vi "Version_4.9_8_on-chip_valves_for25ulSyringe_withModfied_Plunging.vi"() -> ()   [LabVIEW 2020] (continued)
                                n2256 = call "RPickUp(SubVI).vi"("Volume to be picked up"=w2683, "Volume of Syringe"=w2686, "Resolution of PickUP"=w2684, "PickUp Flow Rate (ul/min)"=w2685, "VISA Refnum in"=w2687) -> ()  [unwired: 6 in, 1 out]
                                }
                                frame #1 {
                                n2257 = while {
                                stop <- w2688 stop-if-true
                                n2258 = local read "Stopper that ends \nthe main loops"() -> (w2689:bool)
                                n2259 = local read "VISA Refnum in\nfor Pump"() -> (w2690:refnum<visa-resource-name>)
                                n2260 = case shown="True" w2689 {
                                frame False {
                                }
                                frame True {
                                n2261 = local read "VISA Refnum in\nfor Pump"() -> (w2691:refnum<visa-resource-name>)
                                n2262 = call "HardStopCurrentProcess (SubVI).vi"("VISA Refnum in"=w2691) -> ()  [unwired: 11 in]
                                }
                                }
                                n2263 = call "ProcessCompletionWaiterWithOutPut (SubVI).vi"("VISA Refnum in"=w2690) -> ("Boolean"=w2688:bool)  [unwired: 10 in]
                                }
                                }
                                frame #2 {
                                # "Reads the initial Plunger Position for computing the volume dispensed"
                                n2264 = local read "VISA Refnum in\nfor Pump"() -> (w2693:refnum<visa-resource-name>)
                                n2265 = call "AbsolutePlungerPosition (SubVI).vi"("VISA Refnum in"=w2693) -> ("Plunger Position"=w2692:i32)  [unwired: 10 in]
                                n2266 = local write "Initial Plunger Position"(w2692) -> ()
                                }
                                frame #3 {
                                # "Switch to Port-2"
                                # "Port-2 of the pump is conncted to column-1 of chip"
                                n2267 = local read "VISA Refnum in\nfor Pump"() -> (w2695:refnum<visa-resource-name>)
                                n2268 = call "PortChanger (SubVI).vi"("Port Number"="2", "VISA Refnum in"=w2695) -> ()  [unwired: 10 in]
                                }
                                frame #4 {
                                n2269 = while {
                                stop <- w2696 stop-if-true
                                n2270 = local read "Stopper that ends \nthe main loops"() -> (w2697:bool)
                                n2271 = local read "VISA Refnum in\nfor Pump"() -> (w2698:refnum<visa-resource-name>)
                                n2272 = case shown="True" w2697 {
                                frame False {
                                }
                                frame True {
                                n2273 = local read "VISA Refnum in\nfor Pump"() -> (w2699:refnum<visa-resource-name>)
                                n2274 = call "HardStopCurrentProcess (SubVI).vi"("VISA Refnum in"=w2699) -> ()  [unwired: 11 in]
                                }
                                }
                                n2275 = call "ProcessCompletionWaiterWithOutPut (SubVI).vi"("VISA Refnum in"=w2698) -> ("Boolean"=w2696:bool)  [unwired: 10 in]
                                }
                                }
                                frame #5 {
                                n2276 = local read "Buffer-A1 Dispense\nFlow Rate (ul/min) \nfor Equilibration\nof Column-1"() -> (w2703:dbl)
                                n2277 = local read "Buffer-A1 Pumping\nResolution \nfor Equilibration \nof Column-1"() -> (w2702:T2)
                                n2278 = local read "VISA Refnum in\nfor Pump"() -> (w2705:refnum<visa-resource-name>)
                                n2279 = local write "Pause Data Collection"(FALSE ("Pause Data Collection")) -> ()
                                n2280 = local read "Volume of Syringe"() -> (w2704:dbl)
                                n2281 = call "GoToAbsolutePosition(SubVI).vi"("Absolute Volume Position in Syringe (in ul)"=0.0, "Volume of Syringe"=w2704, "Resolution of Pumping"=w2702, "Flow Rate (ul/min)"=w2703, "VISA Refnum in"=w2705) -> ()  [unwired: 6 in, 1 out]
                                }
                                frame #6 {
                                n2282 = local read "Buffer-A1 Pumping\nResolution \nfor Equilibration \nof Column-1"() -> (w2707:T2)
                                n2283 = local read "VISA Refnum in\nfor Pump"() -> (w2709:refnum<visa-resource-name>)
                                n2284 = local read "Initial Plunger Position"() -> (w2708:dbl)
                                n2285 = local read "Volume of Syringe"() -> (w2706:dbl)
                                n2286 = while {
                                tunnel: w2708 -> [w2716]
                                tunnel: w2709 -> [w2715]
                                tunnel: w2707 -> [w2714]
                                tunnel: w2706 -> [w2713]
                                stop <- w2711 stop-if-true
                                n2287 = stacked-sequence {
                                tunnel: w2716 -> [w2723 _]
                                tunnel: w2715 -> [w2722 w2743]
                                tunnel: w2714 -> [w2721 _]
                                tunnel: w2713 -> [w2720 _]
                                tunnel: [_ w2741] -> w2711
                                frame #0 {
                                n2288 = call "AbsolutePlungerPosition (SubVI).vi"("VISA Refnum in"=w2722) -> ("Plunger Position"=w2719:i32)  [unwired: 10 in]
                                n2289 = case shown="\"Standard Pumping\", Default" w2721 {
                                tunnel: w2723 -> [w2728 w2737]
                                tunnel: w2719 -> [w2729 w2736]
                                tunnel: [w2727 w2734] -> w2718
                                tunnel: w2720 -> [w2726 w2735]
                                frame "Standard Pumping", Default {
                                n2290 = Subtract(x=w2728, y=w2729) -> (x-y=w2725:dbl)
                                n2291 = Absolute Value(x=w2725) -> (abs(x)=w2724:dbl)
                                n2292 = Multiply(x=w2724, y=w2726) -> (x*y=w2731:dbl)
                                n2293 = Divide(x=w2731, y=3000.0) -> (x/y=w2727:dbl)
                                }
                                frame "High Resolution Pumping" {
                                n2294 = Subtract(x=w2737, y=w2736) -> (x-y=w2733:dbl)
                                n2295 = Absolute Value(x=w2733) -> (abs(x)=w2732:dbl)
                                n2296 = Multiply(x=w2732, y=w2735) -> (x*y=w2739:dbl)
                                n2297 = Divide(x=w2739, y=24000.0) -> (x/y=w2734:dbl)
                                }
                                }
                                n2298 = local write "Volume being Injected \nin this process"(w2718) -> ()
                                }
                                frame #1 {
                                n2299 = call "LSPOneStatus (SubVI).vi"("VISA Refnum in"=w2743) -> ("read buffer"=w2745:string)  [unwired: 10 in]
                                n2300 = call <vilib>:"Trim Whitespace.vi"("string"=w2745) -> ("trimmed string"=w2744:string)  [unwired: 1 in]
                                n2301 = local read "Stopper that ends \nthe main loops"() -> (w2740:bool)
                                n2302 = Equal?(x=w2744, y="/0`\u0003") -> (x = y?=w2742:bool)
                                n2303 = Or(x=w2742, y=w2740) -> (x .or. y?=w2741:bool)
                                }
                                }
                                n2304 = Wait (ms)(milliseconds to wait=u32 100) -> ()  [unwired: 1 out]
                                n2305 = local read "Stopper that ends \nthe main loops"() -> (w2710:bool)
                                n2306 = case shown="True" w2710 {
                                frame False {
                                }
                                frame True {
                                n2307 = local read "VISA Refnum in\nfor Pump"() -> (w2717:refnum<visa-resource-name>)
                                n2308 = call "HardStopCurrentProcess (SubVI).vi"("VISA Refnum in"=w2717) -> ()  [unwired: 11 in]
                                }
                                }
                                }
                                }
                                frame #7 {
                                # "Change the pump port back to Buffer-A1"
                                n2309 = local read "VISA Refnum in\nfor Pump"() -> (w2748:refnum<visa-resource-name>)
                                n2310 = local read "Port for \nA1-Equilibriation"() -> (w2747:string)
                                n2311 = local write "Pause Data Collection"(TRUE ("Pause Data Collection")) -> ()
                                n2312 = Wait (ms)(milliseconds to wait=u32 500) -> ()  [unwired: 1 out]
                                n2313 = call "PortChanger (SubVI).vi"("Port Number"=w2747, "VISA Refnum in"=w2748) -> ()  [unwired: 10 in]
                                }
                                frame #8 {
                                n2314 = local read "VISA Refnum in\nfor Pump"() -> (w2751:refnum<visa-resource-name>)
                                n2315 = local write "Volume being Injected \nin this process"(0.0 ("Volume being Injected \nin this process")) -> ()
                                n2316 = call "ProcessCompletionWaiter (SubVI).vi"("VISA Refnum in"=w2751) -> ()  [unwired: 11 in]
                                }
                              }
                            }
                            n2317 = local write "Reminder of the \nVolume to be \nPumped"(w2680) -> ()
                          }
                          frame #6 {
                            n2318 = stacked-sequence {
                              frame #0 {
                                n2319 = local read "Buffer-A1 PickUp \nFlow Rate (ul/min)\nfor Equilibration \nof Column-1"() -> (w2755:dbl)
                                n2320 = local read "Buffer-A1 Pumping\nResolution \nfor Equilibration \nof Column-1"() -> (w2754:T2)
                                n2321 = local read "VISA Refnum in\nfor Pump"() -> (w2757:refnum<visa-resource-name>)
                                n2322 = local read "Reminder of the \nVolume to be \nPumped"() -> (w2753:dbl)
                                n2323 = local read "Volume of Syringe"() -> (w2756:dbl)
                                n2324 = call "RPickUp(SubVI).vi"("Volume to be picked up"=w2753, "Volume of Syringe"=w2756, "Resolution of PickUP"=w2754, "PickUp Flow Rate (ul/min)"=w2755, "VISA Refnum in"=w2757) -> ()  [unwired: 6 in, 1 out]
                              }
                              frame #1 {
                                n2325 = while {
                                stop <- w2758 stop-if-true
                                n2326 = local read "Stopper that ends \nthe main loops"() -> (w2759:bool)
                                n2327 = local read "VISA Refnum in\nfor Pump"() -> (w2760:refnum<visa-resource-name>)
                                n2328 = case shown="True" w2759 {
                                frame False {
                                }
                                frame True {
                                n2329 = local read "VISA Refnum in\nfor Pump"() -> (w2761:refnum<visa-resource-name>)
                                n2330 = call "HardStopCurrentProcess (SubVI).vi"("VISA Refnum in"=w2761) -> ()  [unwired: 11 in]
                                }
                                }
                                n2331 = call "ProcessCompletionWaiterWithOutPut (SubVI).vi"("VISA Refnum in"=w2760) -> ("Boolean"=w2758:bool)  [unwired: 10 in]
                                }
                              }
                              frame #2 {
                                # "Reads the initial Plunger Position for computing the volume dispensed"
                                n2332 = local read "VISA Refnum in\nfor Pump"() -> (w2763:refnum<visa-resource-name>)
                                n2333 = call "AbsolutePlungerPosition (SubVI).vi"("VISA Refnum in"=w2763) -> ("Plunger Position"=w2762:i32)  [unwired: 10 in]
                                n2334 = local write "Initial Plunger Position"(w2762) -> ()
                              }
                              frame #3 {
                                # "Switch to Port-2"
                                # "Port-2 of the pump is conncted to column-1 of chip"
                                n2335 = local read "VISA Refnum in\nfor Pump"() -> (w2765:refnum<visa-resource-name>)
                                n2336 = call "PortChanger (SubVI).vi"("Port Number"="2", "VISA Refnum in"=w2765) -> ()  [unwired: 10 in]
                              }
                              frame #4 {
                                n2337 = while {
                                stop <- w2766 stop-if-true
                                n2338 = local read "Stopper that ends \nthe main loops"() -> (w2767:bool)
                                n2339 = local read "VISA Refnum in\nfor Pump"() -> (w2768:refnum<visa-resource-name>)
                                n2340 = case shown="True" w2767 {
                                frame False {
                                }
                                frame True {
                                n2341 = local read "VISA Refnum in\nfor Pump"() -> (w2769:refnum<visa-resource-name>)
                                n2342 = call "HardStopCurrentProcess (SubVI).vi"("VISA Refnum in"=w2769) -> ()  [unwired: 11 in]
                                }
                                }
                                n2343 = call "ProcessCompletionWaiterWithOutPut (SubVI).vi"("VISA Refnum in"=w2768) -> ("Boolean"=w2766:bool)  [unwired: 10 in]
                                }
                              }
                              frame #5 {
                                n2344 = local read "Buffer-A1 Pumping\nResolution \nfor Equilibration \nof Column-1"() -> (w2772:T2)
                                n2345 = local read "Buffer-A1 Dispense\nFlow Rate (ul/min) \nfor Equilibration\nof Column-1"() -> (w2773:dbl)
                                n2346 = local read "VISA Refnum in\nfor Pump"() -> (w2775:refnum<visa-resource-name>)
                                n2347 = local write "Pause Data Collection"(FALSE ("Pause Data Collection")) -> ()
                                n2348 = local read "Volume of Syringe"() -> (w2774:dbl)
                                n2349 = call "GoToAbsolutePosition(SubVI).vi"("Absolute Volume Position in Syringe (in ul)"=0.0 ("Volume to be Dispensed"), "Volume of Syringe"=w2774, "Resolution of Pumping"=w2772, "Flow Rate (ul/min)"=w2773, "VISA Refnum in"=w2775) -> ()  [unwired: 6 in, 1 out]
                              }
                              frame #6 {
                                n2350 = local read "Buffer-A1 Pumping\nResolution \nfor Equilibration \nof Column-1"() -> (w2777:T2)
                                n2351 = local read "VISA Refnum in\nfor Pump"() -> (w2779:refnum<visa-resource-name>)
                                n2352 = local read "Initial Plunger Position"() -> (w2778:dbl)
                                n2353 = local read "Volume of Syringe"() -> (w2776:dbl)
                                n2354 = while {
                                tunnel: w2778 -> [w2786]
                                tunnel: w2779 -> [w2785]
                                tunnel: w2777 -> [w2784]
                                tunnel: w2776 -> [w2783]
                                stop <- w2781 stop-if-true
                                n2355 = stacked-sequence {
                                tunnel: w2786 -> [w2793 _]
                                tunnel: w2785 -> [w2792 w2813]
                                tunnel: w2784 -> [w2791 _]
                                tunnel: w2783 -> [w2790 _]
                                tunnel: [_ w2811] -> w2781
                                frame #0 {
                                n2356 = call "AbsolutePlungerPosition (SubVI).vi"("VISA Refnum in"=w2792) -> ("Plunger Position"=w2789:i32)  [unwired: 10 in]
                                n2357 = case shown="\"Standard Pumping\", Default" w2791 {
                                tunnel: w2793 -> [w2798 w2807]
                                tunnel: w2789 -> [w2799 w2806]
                                tunnel: [w2797 w2804] -> w2788
                                tunnel: w2790 -> [w2796 w2805]
                                frame "Standard Pumping", Default {
                                n2358 = Subtract(x=w2798, y=w2799) -> (x-y=w2795:dbl)
                                n2359 = Absolute Value(x=w2795) -> (abs(x)=w2794:dbl)
                                n2360 = Multiply(x=w2794, y=w2796) -> (x*y=w2801:dbl)
                                n2361 = Divide(x=w2801, y=3000.0) -> (x/y=w2797:dbl)
                                }
                                frame "High Resolution Pumping" {
                                n2362 = Subtract(x=w2807, y=w2806) -> (x-y=w2803:dbl)
                                n2363 = Absolute Value(x=w2803) -> (abs(x)=w2802:dbl)
                                n2364 = Multiply(x=w2802, y=w2805) -> (x*y=w2809:dbl)
                                n2365 = Divide(x=w2809, y=24000.0) -> (x/y=w2804:dbl)
                                }
                                }
                                n2366 = local write "Volume being Injected \nin this process"(w2788) -> ()
                                }
                                frame #1 {
                                n2367 = call "LSPOneStatus (SubVI).vi"("VISA Refnum in"=w2813) -> ("read buffer"=w2815:string)  [unwired: 10 in]
                                n2368 = call <vilib>:"Trim Whitespace.vi"("string"=w2815) -> ("trimmed string"=w2814:string)  [unwired: 1 in]
                                n2369 = local read "Stopper that ends \nthe main loops"() -> (w2810:bool)
                                n2370 = Equal?(x=w2814, y="/0`\u0003") -> (x = y?=w2812:bool)
                                n2371 = Or(x=w2812, y=w2810) -> (x .or. y?=w2811:bool)
                                }
                                }
                                n2372 = Wait (ms)(milliseconds to wait=u32 100) -> ()  [unwired: 1 out]
                                n2373 = local read "Stopper that ends \nthe main loops"() -> (w2780:bool)
                                n2374 = case shown="True" w2780 {
                                frame False {
                                }
                                frame True {
                                n2375 = local read "VISA Refnum in\nfor Pump"() -> (w2787:refnum<visa-resource-name>)
                                n2376 = call "HardStopCurrentProcess (SubVI).vi"("VISA Refnum in"=w2787) -> ()  [unwired: 11 in]
                                }
                                }
                                }
                              }
                              frame #7 {
                                # "Change the pump port to Buffer-C1 for equilibriation of column-2"
                                n2377 = local read "VISA Refnum in\nfor Pump"() -> (w2818:refnum<visa-resource-name>)
                                n2378 = local read "Port for \nC1-Equilibriation"() -> (w2817:string)
                                n2379 = local write "Pause Data Collection"(TRUE ("Pause Data Collection")) -> ()
                                n2380 = Wait (ms)(milliseconds to wait=u32 500) -> ()  [unwired: 1 out]
                                n2381 = call "PortChanger (SubVI).vi"("Port Number"=w2817, "VISA Refnum in"=w2818) -> ()  [unwired: 10 in]
                              }
                              frame #8 {
                                n2382 = local read "VISA Refnum in\nfor Pump"() -> (w2822:refnum<visa-resource-name>)
                                n2383 = local write "Volume being Injected \nin this process"(0.0 ("Volume being Injected \nin this process")) -> ()
                                n2384 = call "ProcessCompletionWaiter (SubVI).vi"("VISA Refnum in"=w2822) -> ()  [unwired: 11 in]
                                n2385 = local write "Start the Process"(FALSE ("Start the Process")) -> ()
                              }
                            }
                          }
                          frame #7 {
                            # "Clean the tubing with Buffer-C1"
                            n2386 = local read "N-C1"() -> (w2825:i32)
                            n2387 = local write "Equilibriating \nColumn-1"(FALSE ("Equilibriating \nColumn-1")) -> ()
                            n2388 = for {
                              N: w2825 -> [_]
                              n2389 = stacked-sequence {
                                frame #0 {
                                n2390 = local read "Port for \nC1-Equilibriation"() -> (w2828:string)
                                n2391 = local read "VISA Refnum in\nfor Pump"() -> (w2829:refnum<visa-resource-name>)
                                n2392 = call "PortChanger (SubVI).vi"("Port Number"=w2828, "VISA Refnum in"=w2829) -> ()  [unwired: 10 in]
                                }
                                frame #1 {
                                n2393 = local read "VISA Refnum in\nfor Pump"() -> (w2830:refnum<visa-resource-name>)
                                n2394 = call "ProcessCompletionWaiter (SubVI).vi"("VISA Refnum in"=w2830) -> ()  [unwired: 11 in]
                                }
                                frame #2 {
                                n2395 = local read "VISA Refnum in\nfor Pump"() -> (w2835:refnum<visa-resource-name>)
                                n2396 = local read "Apparent Volume\nof Syringe"() -> (w2831:dbl)
                                n2397 = local read "Volume of Syringe"() -> (w2832:dbl)
                                n2398 = call "RPickUp(SubVI).vi"("Volume to be picked up"=w2831, "Volume of Syringe"=w2832, "Resolution of PickUP"=T2."Standard Pumping", "PickUp Flow Rate (ul/min)"=150.0, "VISA Refnum in"=w2835) -> ()  [unwired: 6 in, 1 out]
                                }
                                frame #3 {
                                n2399 = local read "Stopper that ends \nthe main loops"() -> (w2836:bool)
                                n2400 = local read "VISA Refnum in\nfor Pump"() -> (w2837:refnum<visa-resource-name>)
                                n2401 = case shown="True" w2836 {
                                frame False {
                                }
                                frame True {
                                n2402 = local read "VISA Refnum in\nfor Pump"() -> (w2838:refnum<visa-resource-name>)
                                n2403 = call "HardStopCurrentProcess (SubVI).vi"("VISA Refnum in"=w2838) -> ()  [unwired: 11 in]
                                }
                                }
                                n2404 = call "ProcessCompletionWaiter (SubVI).vi"("VISA Refnum in"=w2837) -> ()  [unwired: 11 in]
                                }
                                frame #4 {
                                n2405 = local read "VISA Refnum in\nfor Pump"() -> (w2840:refnum<visa-resource-name>)
                                n2406 = call "PortChanger (SubVI).vi"("Port Number"="1", "VISA Refnum in"=w2840) -> ()  [unwired: 10 in]
                                }
                                frame #5 {
                                n2407 = local read "Stopper that ends \nthe main loops"() -> (w2841:bool)
                                n2408 = local read "VISA Refnum in\nfor Pump"() -> (w2842:refnum<visa-resource-name>)
                                n2409 = case shown="True" w2841 {
                                frame False {
                                }
                                frame True {
                                n2410 = local read "VISA Refnum in\nfor Pump"() -> (w2843:refnum<visa-resource-name>)
                                n2411 = call "HardStopCurrentProcess (SubVI).vi"("VISA Refnum in"=w2843) -> ()  [unwired: 11 in]
                                }
                                }
                                n2412 = call "ProcessCompletionWaiter (SubVI).vi"("VISA Refnum in"=w2842) -> ()  [unwired: 11 in]
                                }
                                frame #6 {
                                n2413 = local read "VISA Refnum in\nfor Pump"() -> (w2848:refnum<visa-resource-name>)
                                n2414 = local read "Volume of Syringe"() -> (w2845:dbl)
                                n2415 = call "GoToAbsolutePosition(SubVI).vi"("Absolute Volume Position in Syringe (in ul)"=0.0 ("Volume to be picked up"), "Volume of Syringe"=w2845, "Resolution of Pumping"=T2."Standard Pumping" ("Resolution of PickUP"), "Flow Rate (ul/min)"=150.0 ("PickUp Flow Rate (ul/min)"), "VISA Refnum in"=w2848) -> ()  [unwired: 6 in, 1 out]
                                }
                                frame #7 {
                                n2416 = local read "Stopper that ends \nthe main loops"() -> (w2849:bool)
                                n2417 = local read "VISA Refnum in\nfor Pump"() -> (w2850:refnum<visa-resource-name>)
                                n2418 = case shown="True" w2849 {
                                frame False {
                                }
                                frame True {
                                n2419 = local read "VISA Refnum in\nfor Pump"() -> (w2851:refnum<visa-resource-name>)
                                n2420 = call "HardStopCurrentProcess (SubVI).vi"("VISA Refnum in"=w2851) -> ()  [unwired: 11 in]
                                }
                                }
                                n2421 = call "ProcessCompletionWaiter (SubVI).vi"("VISA Refnum in"=w2850) -> ()  [unwired: 11 in]
                                }
                              }
                            }
                            n2422 = local write "Pause Data Collection"(TRUE ("Pause Data Collection")) -> ()
                            n2423 = local write "Equilibriating \nColumn-2"(TRUE ("Equilibriating \nColumn-2")) -> ()
                          }
                          frame #8 {
                            n2424 = local read "Buffer-C1 Volume \nto be  Pumped \nfor Equilibration\nof Column-2"() -> (w2855:dbl)
                            n2425 = local read "Apparent Volume\nof Syringe"() -> (w2852:dbl)
                            n2426 = Quotient & Remainder(x=w2855, y=w2852) -> (x-y*floor(x/y)=w2853:dbl, floor(x/y)=w2854:dbl)
                            n2427 = for {
                              N: w2854 -> [_]
                              n2428 = stacked-sequence {
                                frame #0 {
                                n2429 = local read "VISA Refnum in\nfor Pump"() -> (w2857:refnum<visa-resource-name>)
                                n2430 = local read "Port for \nC1-Equilibriation"() -> (w2856:string)
                                n2431 = call "PortChanger (SubVI).vi"("Port Number"=w2856, "VISA Refnum in"=w2857) -> ()  [unwired: 10 in]
                                }
                                frame #1 {
                                n2432 = local read "VISA Refnum in\nfor Pump"() -> (w2858:refnum<visa-resource-name>)
                                n2433 = call "ProcessCompletionWaiter (SubVI).vi"("VISA Refnum in"=w2858) -> ()  [unwired: 11 in]
                                }
                                frame #2 {
                                n2434 = local read "Buffer-C1 PickUp \nFlow Rate (ul/min)\nfor Equilibration \nof Column-2"() -> (w2861:dbl)
                                n2435 = local read "Buffer-C1 Pumping\nResolution \nfor Equilibration \nof Column-2"() -> (w2860:T2)
                                n2436 = local read "VISA Refnum in\nfor Pump"() -> (w2863:refnum<visa-resource-name>)
                                n2437 = local read "Apparent Volume\nof Syringe"() -> (w2859:dbl)
                                n2438 = local read "Volume of Syringe"() -> (w2862:dbl)
                                n2439 = call "RPickUp(SubVI).vi"("Volume to be picked up"=w2859, "Volume of Syringe"=w2862, "Resolution of PickUP"=w2860, "PickUp Flow Rate (ul/min)"=w2861, "VISA Refnum in"=w2863) -> ()  [unwired: 6 in, 1 out]
                                }
                                frame #3 {
                                n2440 = while {
                                stop <- w2864 stop-if-true
                                n2441 = local read "Stopper that ends \nthe main loops"() -> (w2865:bool)
                                n2442 = local read "VISA Refnum in\nfor Pump"() -> (w2866:refnum<visa-resource-name>)
                                n2443 = case shown="True" w2865 {
                                frame False {
                                }
                                frame True {
                                n2444 = local read "VISA Refnum in\nfor Pump"() -> (w2867:refnum<visa-resource-name>)
                                n2445 = call "HardStopCurrentProcess (SubVI).vi"("VISA Refnum in"=w2867) -> ()  [unwired: 11 in]
                                }
                                }
                                n2446 = call "ProcessCompletionWaiterWithOutPut (SubVI).vi"("VISA Refnum in"=w2866) -> ("Boolean"=w2864:bool)  [unwired: 10 in]
                                }
                                }
                                frame #4 {
                                # "Reads the initial Plunger Position for computing the volume dispensed"
                                n2447 = local read "VISA Refnum in\nfor Pump"() -> (w2869:refnum<visa-resource-name>)
                                n2448 = call "AbsolutePlungerPosition (SubVI).vi"("VISA Refnum in"=w2869) -> ("Plunger Position"=w2868:i32)  [unwired: 10 in]
                                n2449 = local write "Initial Plunger Position"(w2868) -> ()
                                }
                                frame #5 {
                                # "Switch to Port-10"
                                # "Port-10 of the pump is conncted to column-2 of chip"
                                n2450 = local read "VISA Refnum in\nfor Pump"() -> (w2871:refnum<visa-resource-name>)
                                n2451 = call "PortChanger (SubVI).vi"("Port Number"="10", "VISA Refnum in"=w2871) -> ()  [unwired: 10 in]
                                }
                                frame #6 {
                                n2452 = while {
                                stop <- w2872 stop-if-true
                                n2453 = local read "Stopper that ends \nthe main loops"() -> (w2873:bool)
                                n2454 = local read "VISA Refnum in\nfor Pump"() -> (w2874:refnum<visa-resource-name>)
                                n2455 = case shown="True" w2873 {
                                frame False {
                                }
                                frame True {
                                n2456 = local read "VISA Refnum in\nfor Pump"() -> (w2875:refnum<visa-resource-name>)
                                n2457 = call "HardStopCurrentProcess (SubVI).vi"("VISA Refnum in"=w2875) -> ()  [unwired: 11 in]
                                }
                                }
                                n2458 = call "ProcessCompletionWaiterWithOutPut (SubVI).vi"("VISA Refnum in"=w2874) -> ("Boolean"=w2872:bool)  [unwired: 10 in]
                                }
                                }
                                frame #7 {
                                # "Buffer-C pumped for column non-interference"
                                # "Keeps the AMF valve after column-1 open and valve after column-2 closed"
                                n2459 = local read "Buffer-C1 Dispense\nFlow Rate (ul/min) \nfor Equilibration\nof Column-2"() -> (w2888:dbl)
                                n2460 = local read "Buffer-C1 Pumping\nResolution \nfor Equilibration \nof Column-2"() -> (w2887:T2)
                                n2461 = local read "VISA Refnum in\nfor Pump"() -> (w2890:refnum<visa-resource-name>)
                                n2462 = local write "Pause Data Collection"(FALSE ("Pause Data Collection")) -> ()
                                n2463 = local read "Volume of Syringe"() -> (w2889:dbl)
                                n2464 = call "GoToAbsolutePosition(SubVI).vi"("Absolute Volume Position in Syringe (in ul)"=0.0, "Volume of Syringe"=w2889, "Resolution of Pumping"=w2887, "Flow Rate (ul/min)"=w2888, "VISA Refnum in"=w2890) -> ()  [unwired: 6 in, 1 out]
                                n2465 = local write "Valve V1 Open"(FALSE ("Valve V1 Open")) -> ()
                                n2466 = local write "Valve V2 Open"(TRUE ("Valve V2 Open")) -> ()
                                n2467 = local write "Valve V4 Open"(FALSE ("Valve V4 Open")) -> ()
                                n2468 = local write "Valve V3 Open"(TRUE ("Valve V3 Open")) -> ()
                                n2469 = local read "VISA Refnum in\nfor Valve"() -> (w2881:refnum<visa-resource-name>)
                                n2470 = local read "External Valve \nOPEN"() -> (w2880:string)
                                n2471 = local write "Valve V5 Open"(FALSE ("Valve V5 Open")) -> ()
                                n2472 = local write "Valve V6 Open"(FALSE ("Valve V6 Open")) -> ()
                                n2473 = local write "Valve V7 Open"(FALSE ("Valve V7 Open")) -> ()
                                n2474 = call "PortChanger_Valve (SubVI).vi"("Port Number"=w2880, "VISA Refnum in"=w2881) -> ()  [unwired: 10 in]
                                }
                                frame #8 {
                                n2475 = local read "Buffer-C1 Pumping\nResolution \nfor Equilibration \nof Column-2"() -> (w2892:T2)
                                n2476 = local read "VISA Refnum in\nfor Pump"() -> (w2894:refnum<visa-resource-name>)
                                n2477 = local read "Initial Plunger Position"() -> (w2893:dbl)
                                n2478 = local read "Volume of Syringe"() -> (w2891:dbl)
                                n2479 = while {
                                tunnel: w2893 -> [w2901]
                                tunnel: w2894 -> [w2900]
                                tunnel: w2892 -> [w2899]
                                tunnel: w2891 -> [w2898]
                                stop <- w2896 stop-if-true
                                n2480 = stacked-sequence {
                                tunnel: w2901 -> [w2908 _]
                                tunnel: w2900 -> [w2907 w2932]
                                tunnel: w2899 -> [w2906 _]
                                tunnel: w2898 -> [w2905 _]
                                tunnel: [_ w2930] -> w2896
                                frame #0 {
                                n2481 = call "AbsolutePlungerPosition (SubVI).vi"("VISA Refnum in"=w2907) -> ("Plunger Position"=w2904:i32)  [unwired: 10 in]
                                n2482 = case shown="\"Standard Pumping\", Default" w2906 {
                                tunnel: w2908 -> [w2913 w2922]
                                tunnel: w2904 -> [w2914 w2921]
                                tunnel: [w2912 w2919] -> w2903
                                tunnel: w2905 -> [w2911 w2920]
                                frame "Standard Pumping", Default {
                                n2483 = Subtract(x=w2913, y=w2914) -> (x-y=w2910:dbl)
                                n2484 = Absolute Value(x=w2910) -> (abs(x)=w2909:dbl)
                                n2485 = Multiply(x=w2909, y=w2911) -> (x*y=w2916:dbl)
                                n2486 = Divide(x=w2916, y=3000.0) -> (x/y=w2912:dbl)
                                }
                                frame "High Resolution Pumping" {
                                n2487 = Subtract(x=w2922, y=w2921) -> (x-y=w2918:dbl)
                                n2488 = Absolute Value(x=w2918) -> (abs(x)=w2917:dbl)
                                n2489 = Multiply(x=w2917, y=w2920) -> (x*y=w2924:dbl)
                                n2490 = Divide(x=w2924, y=24000.0) -> (x/y=w2919:dbl)
                                }
                                }
                                n2491 = local write "Volume being Injected \nin this process"(w2903) -> ()
                                }
                                frame #1 {
                                n2492 = local read "Buffer-C Volume \nto be Pumped for\nColumn \nnon-interference"() -> (w2928:dbl)
                                n2493 = local read "Volume being Injected \nin this process"() -> (w2929:dbl)
                                n2494 = local read "Stopper that ends \nthe main loops"() -> (w2927:bool)
                                n2495 = call "LSPOneStatus (SubVI).vi"("VISA Refnum in"=w2932) -> ("read buffer"=w2934:string)  [unwired: 10 in]
                                n2496 = call <vilib>:"Trim Whitespace.vi"("string"=w2934) -> ("trimmed string"=w2933:string)  [unwired: 1 in]
                                n2497 = Equal?(x=w2933, y="/0`\u0003") -> (x = y?=w2931:bool)
                                n2498 = Greater Or Equal?(x=w2929, y=w2928) -> (x >= y?=w2926:bool)
                                n2499 = Or(x=w2927, y=w2926) -> (x .or. y?=w2925:bool)
                                n2500 = Or(x=w2931, y=w2925) -> (x .or. y?=w2930:bool)
                                }
                                }
                                n2501 = Wait (ms)(milliseconds to wait=u32 100) -> ()  [unwired: 1 out]
                                n2502 = local read "Stopper that ends \nthe main loops"() -> (w2895:bool)
                                n2503 = case shown="True" w2895 {
                                frame False {
                                }
                                frame True {
                                n2504 = local read "VISA Refnum in\nfor Pump"() -> (w2902:refnum<visa-resource-name>)
                                n2505 = call "HardStopCurrentProcess (SubVI).vi"("VISA Refnum in"=w2902) -> ()  [unwired: 11 in]
                                }
                                }
                                }
                                }
                                frame #9 {
                                # "Keeps the AMF valve after column-1 closed and valve after column-2 open"
                                n2506 = local read "VISA Refnum in\nfor Valve"() -> (w2940:refnum<visa-resource-name>)
                                n2507 = local read "External Valve \nCLOSED"() -> (w2939:string)
                                n2508 = local write "Valve V3 Open"(FALSE ("Valve V3 Open")) -> ()
                                n2509 = local write "Valve V2 Open"(FALSE ("Valve V2 Open")) -> ()
                                n2510 = local write "Valve V4 Open"(TRUE ("Valve V1 Open")) -> ()
                                n2511 = local write "Valve V1 Open"(FALSE ("Valve V1 Open")) -> ()
                                n2512 = call "PortChanger_Valve (SubVI).vi"("Port Number"=w2939, "VISA Refnum in"=w2940) -> ()  [unwired: 10 in]
                                n2513 = local write "Valve V5 Open"(TRUE ("Valve V4 Open")) -> ()
                                n2514 = local write "Valve V7 Open"(TRUE ("Valve V6 Open")) -> ()
                                n2515 = local write "Valve V6 Open"(FALSE ("Valve V6 Open")) -> ()
                                }
                                frame #10 {
                                n2516 = local read "Buffer-C1 Pumping\nResolution \nfor Equilibration \nof Column-2"() -> (w2946:T2)
                                n2517 = local read "VISA Refnum in\nfor Pump"() -> (w2948:refnum<visa-resource-name>)
                                n2518 = local read "Initial Plunger Position"() -> (w2947:dbl)
                                n2519 = local read "Volume of Syringe"() -> (w2945:dbl)
                                n2520 = while {
                                tunnel: w2947 -> [w2955]
                                tunnel: w2948 -> [w2954]
                                tunnel: w2946 -> [w2953]
                                tunnel: w2945 -> [w2952]
                                stop <- w2950 stop-if-true
                                n2521 = stacked-sequence {
                                tunnel: w2955 -> [w2962 _]
                                tunnel: w2954 -> [w2961 w2982]
                                tunnel: w2953 -> [w2960 _]
                                tunnel: w2952 -> [w2959 _]
                                tunnel: [_ w2980] -> w2950
                                frame #0 {
                                n2522 = call "AbsolutePlungerPosition (SubVI).vi"("VISA Refnum in"=w2961) -> ("Plunger Position"=w2958:i32)  [unwired: 10 in]
                                n2523 = case shown="\"Standard Pumping\", Default" w2960 {
                                tunnel: w2962 -> [w2967 w2976]
                                tunnel: w2958 -> [w2968 w2975]
                                tunnel: [w2966 w2973] -> w2957
                                tunnel: w2959 -> [w2965 w2974]
                                frame "Standard Pumping", Default {
                                n2524 = Subtract(x=w2967, y=w2968) -> (x-y=w2964:dbl)
                                n2525 = Absolute Value(x=w2964) -> (abs(x)=w2963:dbl)
                                n2526 = Multiply(x=w2963, y=w2965) -> (x*y=w2970:dbl)
                                n2527 = Divide(x=w2970, y=3000.0) -> (x/y=w2966:dbl)
                                }
                                frame "High Resolution Pumping" {
                                n2528 = Subtract(x=w2976, y=w2975) -> (x-y=w2972:dbl)
                                n2529 = Absolute Value(x=w2972) -> (abs(x)=w2971:dbl)
                                n2530 = Multiply(x=w2971, y=w2974) -> (x*y=w2978:dbl)
                                n2531 = Divide(x=w2978, y=24000.0) -> (x/y=w2973:dbl)
                                }
                                }
                                n2532 = local write "Volume being Injected \nin this process"(w2957) -> ()
                                }
                                frame #1 {
                                n2533 = local read "Stopper that ends \nthe main loops"() -> (w2979:bool)
                                n2534 = call "LSPOneStatus (SubVI).vi"("VISA Refnum in"=w2982) -> ("read buffer"=w2984:string)  [unwired: 10 in]
                                n2535 = call <vilib>:"Trim Whitespace.vi"("string"=w2984) -> ("trimmed string"=w2983:string)  [unwired: 1 in]
                                n2536 = Equal?(x=w2983, y="/0`\u0003") -> (x = y?=w2981:bool)
                                n2537 = Or(x=w2981, y=w2979) -> (x .or. y?=w2980:bool)
                                }
                                }
                                n2538 = Wait (ms)(milliseconds to wait=u32 100) -> ()  [unwired: 1 out]
                                n2539 = local read "Stopper that ends \nthe main loops"() -> (w2949:bool)
                                n2540 = case shown="True" w2949 {
                                frame False {
                                }
                                frame True {
                                n2541 = local read "VISA Refnum in\nfor Pump"() -> (w2956:refnum<visa-resource-name>)
                                n2542 = call "HardStopCurrentProcess (SubVI).vi"("VISA Refnum in"=w2956) -> ()  [unwired: 11 in]
                                }
                                }
                                }
                                }
                                frame #11 {
                                # "Change the pump port back to Buffer-C1"
                                n2543 = local read "VISA Refnum in\nfor Pump"() -> (w2987:refnum<visa-resource-name>)
                                n2544 = local read "Port for \nC1-Equilibriation"() -> (w2986:string)
                                n2545 = local write "Pause Data Collection"(TRUE ("Pause Data Collection")) -> ()
                                n2546 = Wait (ms)(milliseconds to wait=u32 500) -> ()  [unwired: 1 out]
                                n2547 = call "PortChanger (SubVI).vi"("Port Number"=w2986, "VISA Refnum in"=w2987) -> ()  [unwired: 10 in]
                                }
                                frame #12 {
                                n2548 = local read "VISA Refnum in\nfor Pump"() -> (w2990:refnum<visa-resource-name>)
                                n2549 = local write "Volume being Injected \nin this process"(0.0 ("Volume being Injected \nin this process")) -> ()
                                n2550 = call "ProcessCompletionWaiter (SubVI).vi"("VISA Refnum in"=w2990) -> ()  [unwired: 11 in]
                                }
                              }
                            }
                            n2551 = local write "Reminder of the \nVolume to be \nPumped"(w2853) -> ()
                          }
                          frame #9 {
                            n2552 = stacked-sequence {
                              frame #0 {
                                n2553 = local read "Buffer-C1 PickUp \nFlow Rate (ul/min)\nfor Equilibration \nof Column-2"() -> (w2994:dbl)
                                n2554 = local read "Buffer-C1 Pumping\nResolution \nfor Equilibration \nof Column-2"() -> (w2993:T2)
                                n2555 = local read "VISA Refnum in\nfor Pump"() -> (w2996:refnum<visa-resource-name>)
                                n2556 = local read "Reminder of the \nVolume to be \nPumped"() -> (w2992:dbl)
                                n2557 = local read "Volume of Syringe"() -> (w2995:dbl)
                                n2558 = call "RPickUp(SubVI).vi"("Volume to be picked up"=w2992, "Volume of Syringe"=w2995, "Resolution of PickUP"=w2993, "PickUp Flow Rate (ul/min)"=w2994, "VISA Refnum in"=w2996) -> ()  [unwired: 6 in, 1 out]
                              }
                              frame #1 {
                                n2559 = while {
                                stop <- w2997 stop-if-true
                                n2560 = local read "Stopper that ends \nthe main loops"() -> (w2998:bool)
                                n2561 = local read "VISA Refnum in\nfor Pump"() -> (w2999:refnum<visa-resource-name>)
                                n2562 = case shown="True" w2998 {
                                frame False {
                                }
                                frame True {
                                n2563 = local read "VISA Refnum in\nfor Pump"() -> (w3000:refnum<visa-resource-name>)
                                n2564 = call "HardStopCurrentProcess (SubVI).vi"("VISA Refnum in"=w3000) -> ()  [unwired: 11 in]
                                }
                                }
                                n2565 = call "ProcessCompletionWaiterWithOutPut (SubVI).vi"("VISA Refnum in"=w2999) -> ("Boolean"=w2997:bool)  [unwired: 10 in]
                                }
                              }
                              frame #2 {
                                # "Reads the initial Plunger Position for computing the volume dispensed"
                                n2566 = local read "VISA Refnum in\nfor Pump"() -> (w3002:refnum<visa-resource-name>)
                                n2567 = call "AbsolutePlungerPosition (SubVI).vi"("VISA Refnum in"=w3002) -> ("Plunger Position"=w3001:i32)  [unwired: 10 in]
                                n2568 = local write "Initial Plunger Position"(w3001) -> ()
                              }
                              frame #3 {
                                # "Switch to Port-10"
                                # "Port-10 of the pump is conncted to column-2 of chip"
                                n2569 = local read "VISA Refnum in\nfor Pump"() -> (w3004:refnum<visa-resource-name>)
                                n2570 = call "PortChanger (SubVI).vi"("Port Number"="10", "VISA Refnum in"=w3004) -> ()  [unwired: 10 in]
                              }
                              frame #4 {
                                n2571 = while {
                                stop <- w3005 stop-if-true
                                n2572 = local read "Stopper that ends \nthe main loops"() -> (w3006:bool)
                                n2573 = local read "VISA Refnum in\nfor Pump"() -> (w3007:refnum<visa-resource-name>)
                                n2574 = case shown="True" w3006 {
                                frame False {
                                }
                                frame True {
                                n2575 = local read "VISA Refnum in\nfor Pump"() -> (w3008:refnum<visa-resource-name>)
                                n2576 = call "HardStopCurrentProcess (SubVI).vi"("VISA Refnum in"=w3008) -> ()  [unwired: 11 in]
                                }
                                }
                                n2577 = call "ProcessCompletionWaiterWithOutPut (SubVI).vi"("VISA Refnum in"=w3007) -> ("Boolean"=w3005:bool)  [unwired: 10 in]
                                }
                              }
                              frame #5 {
                                # "Keeps the AMF valve after column-1 open and valve after column-2 closed"
                                n2578 = local read "Buffer-C1 Dispense\nFlow Rate (ul/min) \nfor Equilibration\nof Column-2"() -> (w3021:dbl)
                                n2579 = local read "Buffer-C1 Pumping\nResolution \nfor Equilibration \nof Column-2"() -> (w3020:T2)
                                n2580 = local read "VISA Refnum in\nfor Pump"() -> (w3023:refnum<visa-resource-name>)
                                n2581 = local write "Pause Data Collection"(FALSE ("Pause Data Collection")) -> ()
                                n2582 = local read "Volume of Syringe"() -> (w3022:dbl)
                                n2583 = call "GoToAbsolutePosition(SubVI).vi"("Absolute Volume Position in Syringe (in ul)"=0.0, "Volume of Syringe"=w3022, "Resolution of Pumping"=w3020, "Flow Rate (ul/min)"=w3021, "VISA Refnum in"=w3023) -> ()  [unwired: 6 in, 1 out]
                                n2584 = local read "VISA Refnum in\nfor Valve"() -> (w3013:refnum<visa-resource-name>)
                                n2585 = local write "Valve V1 Open"(FALSE ("Valve V1 Open")) -> ()
                                n2586 = local write "Valve V2 Open"(TRUE ("Valve V2 Open")) -> ()
                                n2587 = local write "Valve V3 Open"(TRUE ("Valve V3 Open")) -> ()
                                n2588 = local write "Valve V4 Open"(FALSE ("Affinity On")) -> ()
                                n2589 = local read "External Valve \nOPEN"() -> (w3012:string)
                                n2590 = local write "Valve V5 Open"(FALSE ("Valve V5 Open")) -> ()
                                n2591 = local write "Valve V6 Open"(FALSE ("Valve V6 Open")) -> ()
                                n2592 = local write "Valve V7 Open"(FALSE ("Valve V7 Open")) -> ()
                                n2593 = call "PortChanger_Valve (SubVI).vi"("Port Number"=w3012, "VISA Refnum in"=w3013) -> ()  [unwired: 10 in]
                              }
                              frame #6 {
                                n2594 = local read "Buffer-C1 Pumping\nResolution \nfor Equilibration \nof Column-2"() -> (w3025:T2)
                                n2595 = local read "VISA Refnum in\nfor Pump"() -> (w3027:refnum<visa-resource-name>)
                                n2596 = local read "Initial Plunger Position"() -> (w3026:dbl)
                                n2597 = local read "Volume of Syringe"() -> (w3024:dbl)
                                n2598 = while {
                                tunnel: w3026 -> [w3034]
                                tunnel: w3027 -> [w3033]
                                tunnel: w3025 -> [w3032]
                                tunnel: w3024 -> [w3031]
                                stop <- w3029 stop-if-true
                                n2599 = stacked-sequence {
                                tunnel: w3034 -> [w3041 _]
                                tunnel: w3033 -> [w3040 w3065]
                                tunnel: w3032 -> [w3039 _]
                                tunnel: w3031 -> [w3038 _]
                                tunnel: [_ w3063] -> w3029
                                frame #0 {
                                n2600 = call "AbsolutePlungerPosition (SubVI).vi"("VISA Refnum in"=w3040) -> ("Plunger Position"=w3037:i32)  [unwired: 10 in]
                                n2601 = case shown="\"Standard Pumping\", Default" w3039 {
                                tunnel: w3041 -> [w3046 w3055]
                                tunnel: w3037 -> [w3047 w3054]
                                tunnel: [w3045 w3052] -> w3036
                                tunnel: w3038 -> [w3044 w3053]
                                frame "Standard Pumping", Default {
                                n2602 = Subtract(x=w3046, y=w3047) -> (x-y=w3043:dbl)
                                n2603 = Absolute Value(x=w3043) -> (abs(x)=w3042:dbl)
                                n2604 = Multiply(x=w3042, y=w3044) -> (x*y=w3049:dbl)
                                n2605 = Divide(x=w3049, y=3000.0) -> (x/y=w3045:dbl)
                                }
                                frame "High Resolution Pumping" {
                                n2606 = Subtract(x=w3055, y=w3054) -> (x-y=w3051:dbl)
                                n2607 = Absolute Value(x=w3051) -> (abs(x)=w3050:dbl)
                                n2608 = Multiply(x=w3050, y=w3053) -> (x*y=w3057:dbl)
                                n2609 = Divide(x=w3057, y=24000.0) -> (x/y=w3052:dbl)
                                }
                                }
                                n2610 = local write "Volume being Injected \nin this process"(w3036) -> ()
                                }
                                frame #1 {
                                n2611 = local read "Buffer-C Volume \nto be Pumped for\nColumn \nnon-interference"() -> (w3061:dbl)
                                n2612 = local read "Volume being Injected \nin this process"() -> (w3062:dbl)
                                n2613 = local read "Stopper that ends \nthe main loops"() -> (w3060:bool)
                                n2614 = call "LSPOneStatus (SubVI).vi"("VISA Refnum in"=w3065) -> ("read buffer"=w3067:string)  [unwired: 10 in]
                                n2615 = call <vilib>:"Trim Whitespace.vi"("string"=w3067) -> ("trimmed string"=w3066:string)  [unwired: 1 in]
                                n2616 = Equal?(x=w3066, y="/0`\u0003") -> (x = y?=w3064:bool)
                                n2617 = Greater Or Equal?(x=w3062, y=w3061) -> (x >= y?=w3059:bool)
                                n2618 = Or(x=w3060, y=w3059) -> (x .or. y?=w3058:bool)
                                n2619 = Or(x=w3064, y=w3058) -> (x .or. y?=w3063:bool)
                                }
                                }
                                n2620 = Wait (ms)(milliseconds to wait=u32 100) -> ()  [unwired: 1 out]
                                n2621 = local read "Stopper that ends \nthe main loops"() -> (w3028:bool)
                                n2622 = case shown="True" w3028 {
                                frame False {
                                }
                                frame True {
                                n2623 = local read "VISA Refnum in\nfor Pump"() -> (w3035:refnum<visa-resource-name>)
                                n2624 = call "HardStopCurrentProcess (SubVI).vi"("VISA Refnum in"=w3035) -> ()  [unwired: 11 in]
                                }
                                }
                                }
                              }
                              frame #7 {
                                # "Keeps the AMF valve after column-1 closed and valve after column-2 open"
                                n2625 = local read "VISA Refnum in\nfor Valve"() -> (w3073:refnum<visa-resource-name>)
                                n2626 = local read "External Valve \nCLOSED"() -> (w3072:string)
                                n2627 = local write "Valve V4 Open"(TRUE ("Valve V4 Open")) -> ()
                                n2628 = local write "Valve V1 Open"(FALSE ("Valve V1 Open")) -> ()
                                n2629 = local write "Valve V2 Open"(FALSE ("Valve V2 Open")) -> ()
                                n2630 = local write "Valve V3 Open"(FALSE ("Valve V3 Open")) -> ()
                                n2631 = call "PortChanger_Valve (SubVI).vi"("Port Number"=w3072, "VISA Refnum in"=w3073) -> ()  [unwired: 10 in]
                                n2632 = local write "Valve V7 Open"(TRUE ("Valve V7 Open")) -> ()
                                n2633 = local write "Valve V5 Open"(TRUE ("Valve V5 Open")) -> ()
                                n2634 = local write "Valve V6 Open"(TRUE ("Valve V6 Open")) -> ()
                              }
                              frame #8 {
                                n2635 = local read "Buffer-C1 Pumping\nResolution \nfor Equilibration \nof Column-2"() -> (w3079:T2)
                                n2636 = local read "VISA Refnum in\nfor Pump"() -> (w3081:refnum<visa-resource-name>)
                                n2637 = local read "Initial Plunger Position"() -> (w3080:dbl)
                                n2638 = local read "Volume of Syringe"() -> (w3078:dbl)
                                n2639 = while {
                                tunnel: w3080 -> [w3088]
                                tunnel: w3081 -> [w3087]
                                tunnel: w3079 -> [w3086]
                                tunnel: w3078 -> [w3085]
                                stop <- w3083 stop-if-true
                                n2640 = stacked-sequence {
                                tunnel: w3088 -> [w3095 _]
                                tunnel: w3087 -> [w3094 w3115]
                                tunnel: w3086 -> [w3093 _]
                                tunnel: w3085 -> [w3092 _]
                                tunnel: [_ w3113] -> w3083
                                frame #0 {
                                n2641 = call "AbsolutePlungerPosition (SubVI).vi"("VISA Refnum in"=w3094) -> ("Plunger Position"=w3091:i32)  [unwired: 10 in]
                                n2642 = case shown="\"Standard Pumping\", Default" w3093 {
                                tunnel: w3095 -> [w3100 w3109]
                                tunnel: w3091 -> [w3101 w3108]
                                tunnel: [w3099 w3106] -> w3090
                                tunnel: w3092 -> [w3098 w3107]
                                frame "Standard Pumping", Default {
                                n2643 = Subtract(x=w3100, y=w3101) -> (x-y=w3097:dbl)
                                n2644 = Absolute Value(x=w3097) -> (abs(x)=w3096:dbl)
                                n2645 = Multiply(x=w3096, y=w3098) -> (x*y=w3103:dbl)
                                n2646 = Divide(x=w3103, y=3000.0) -> (x/y=w3099:dbl)
                                }
                                frame "High Resolution Pumping" {
                                n2647 = Subtract(x=w3109, y=w3108) -> (x-y=w3105:dbl)
                                n2648 = Absolute Value(x=w3105) -> (abs(x)=w3104:dbl)
                                n2649 = Multiply(x=w3104, y=w3107) -> (x*y=w3111:dbl)
                                n2650 = Divide(x=w3111, y=24000.0) -> (x/y=w3106:dbl)
                                }
                                }
                                n2651 = local write "Volume being Injected \nin this process"(w3090) -> ()
                                }
                                frame #1 {
                                n2652 = local read "Stopper that ends \nthe main loops"() -> (w3112:bool)
                                n2653 = call "LSPOneStatus (SubVI).vi"("VISA Refnum in"=w3115) -> ("read buffer"=w3117:string)  [unwired: 10 in]
                                n2654 = call <vilib>:"Trim Whitespace.vi"("string"=w3117) -> ("trimmed string"=w3116:string)  [unwired: 1 in]
                                n2655 = Equal?(x=w3116, y="/0`\u0003") -> (x = y?=w3114:bool)
                                n2656 = Or(x=w3114, y=w3112) -> (x .or. y?=w3113:bool)
                                }
                                }
                                n2657 = Wait (ms)(milliseconds to wait=u32 100) -> ()  [unwired: 1 out]
                                n2658 = local read "Stopper that ends \nthe main loops"() -> (w3082:bool)
                                n2659 = case shown="True" w3082 {
                                frame False {
                                }
                                frame True {
                                n2660 = local read "VISA Refnum in\nfor Pump"() -> (w3089:refnum<visa-resource-name>)
                                n2661 = call "HardStopCurrentProcess (SubVI).vi"("VISA Refnum in"=w3089) -> ()  [unwired: 11 in]
                                }
                                }
                                }
                              }
                              frame #9 {
                                n2662 = local write "Pause Data Collection"(TRUE ("Pause Data Collection")) -> ()
                                n2663 = Wait (ms)(milliseconds to wait=u32 500) -> ()  [unwired: 1 out]
                              }
                              frame #10 {
                                n2664 = local write "Volume being Injected \nin this process"(0.0 ("Volume being Injected \nin this process")) -> ()
                                n2665 = local write "Start the Process"(FALSE ("Start the Process")) -> ()
                              }
                            }
                          }
                          frame #10 {
                            # "Clean the tubing with Sample"
                            n2666 = local read "N-S"() -> (w3123:i32)
                            n2667 = for {
                              N: w3123 -> [_]
                              n2668 = stacked-sequence {
                                frame #0 {
                                n2669 = local read "VISA Refnum in\nfor Pump"() -> (w3126:refnum<visa-resource-name>)
                                n2670 = local read "Port for \nSample"() -> (w3125:string)
                                n2671 = call "PortChanger (SubVI).vi"("Port Number"=w3125, "VISA Refnum in"=w3126) -> ()  [unwired: 10 in]
                                }
                                frame #1 {
                                n2672 = local read "VISA Refnum in\nfor Pump"() -> (w3127:refnum<visa-resource-name>)
                                n2673 = call "ProcessCompletionWaiter (SubVI).vi"("VISA Refnum in"=w3127) -> ()  [unwired: 11 in]
                                }
                                frame #2 {
                                n2674 = local read "VISA Refnum in\nfor Pump"() -> (w3132:refnum<visa-resource-name>)
                                n2675 = local read "Sample PickUp \nFlow Rate (ul/min)"() -> (w3129:dbl)
                                n2676 = local read "V-S"() -> (w3128:dbl)
                                n2677 = local read "Volume of Syringe"() -> (w3130:dbl)
                                n2678 = call "RPickUp(SubVI).vi"("Volume to be picked up"=w3128, "Volume of Syringe"=w3130, "Resolution of PickUP"=T2."Standard Pumping", "PickUp Flow Rate (ul/min)"=w3129, "VISA Refnum in"=w3132) -> ()  [unwired: 6 in, 1 out]
                                }
                                frame #3 {
                                n2679 = local read "Stopper that ends \nthe main loops"() -> (w3133:bool)
                                n2680 = local read "VISA Refnum in\nfor Pump"() -> (w3134:refnum<visa-resource-name>)
                                n2681 = case shown="True" w3133 {
                                frame False {
                                }
                                frame True {
                                n2682 = local read "VISA Refnum in\nfor Pump"() -> (w3135:refnum<visa-resource-name>)
                                n2683 = call "HardStopCurrentProcess (SubVI).vi"("VISA Refnum in"=w3135) -> ()  [unwired: 11 in]
                                }
                                }
                                n2684 = call "ProcessCompletionWaiter (SubVI).vi"("VISA Refnum in"=w3134) -> ()  [unwired: 11 in]
                                }
                                frame #4 {
                                n2685 = local read "VISA Refnum in\nfor Pump"() -> (w3137:refnum<visa-resource-name>)
                                n2686 = call "PortChanger (SubVI).vi"("Port Number"="1", "VISA Refnum in"=w3137) -> ()  [unwired: 10 in]
                                }
                                frame #5 {
                                n2687 = local read "Stopper that ends \nthe main loops"() -> (w3138:bool)
                                n2688 = local read "VISA Refnum in\nfor Pump"() -> (w3139:refnum<visa-resource-name>)
                                n2689 = case shown="True" w3138 {
                                frame False {
                                }
                                frame True {
                                n2690 = local read "VISA Refnum in\nfor Pump"() -> (w3140:refnum<visa-resource-name>)
                                n2691 = call "HardStopCurrentProcess (SubVI).vi"("VISA Refnum in"=w3140) -> ()  [unwired: 11 in]
                                }
                                }
                                n2692 = call "ProcessCompletionWaiter (SubVI).vi"("VISA Refnum in"=w3139) -> ()  [unwired: 11 in]
                                }
                                frame #6 {
                                n2693 = local read "VISA Refnum in\nfor Pump"() -> (w3145:refnum<visa-resource-name>)
                                n2694 = local read "Volume of Syringe"() -> (w3142:dbl)
                                n2695 = call "GoToAbsolutePosition(SubVI).vi"("Absolute Volume Position in Syringe (in ul)"=0.0 ("Volume to be picked up"), "Volume of Syringe"=w3142, "Resolution of Pumping"=T2."Standard Pumping" ("Resolution of PickUP"), "Flow Rate (ul/min)"=150.0 ("PickUp Flow Rate (ul/min)"), "VISA Refnum in"=w3145) -> ()  [unwired: 6 in, 1 out]
                                }
                                frame #7 {
                                n2696 = local read "Stopper that ends \nthe main loops"() -> (w3146:bool)
                                n2697 = local read "VISA Refnum in\nfor Pump"() -> (w3147:refnum<visa-resource-name>)
                                n2698 = case shown="True" w3146 {
                                frame False {
                                }
                                frame True {
                                n2699 = local read "VISA Refnum in\nfor Pump"() -> (w3148:refnum<visa-resource-name>)
                                n2700 = call "HardStopCurrentProcess (SubVI).vi"("VISA Refnum in"=w3148) -> ()  [unwired: 11 in]
                                }
                                }
                                n2701 = call "ProcessCompletionWaiter (SubVI).vi"("VISA Refnum in"=w3147) -> ()  [unwired: 11 in]
                                }
                              }
                              n2702 = local write "Pause Data Collection"(TRUE ("Pause Data Collection")) -> ()
                            }
                          }
                        }
                      }
                      frame #1 {
                        # "Pump Purified Sample into Column-2"
                        n2703 = stacked-sequence {
                          frame #0 {
                            # "Switch to Port-3"
                            # "Port-3 of pump is connected to Sample"
                            n2704 = local read "VISA Refnum in\nfor Pump"() -> (w3153:refnum<visa-resource-name>)
                            n2705 = local read "Port for \nSample"() -> (w3152:string)
                            n2706 = call "PortChanger (SubVI).vi"("Port Number"=w3152, "VISA Refnum in"=w3153) -> ()  [unwired: 10 in]
                          }
                          frame #1 {
                            n2707 = local read "VISA Refnum in\nfor Pump"() -> (w3154:refnum<visa-resource-name>)
                            n2708 = call "ProcessCompletionWaiter (SubVI).vi"("VISA Refnum in"=w3154) -> ()  [unwired: 11 in]
                          }
                          frame #2 {
                            # "V4 is open"
                            # "V1, V2 and V3 are closed"
                            n2709 = local read "VISA Refnum in\nfor Valve"() -> (w3159:refnum<visa-resource-name>)
                            n2710 = local read "External Valve \nCLOSED"() -> (w3158:string)
                            n2711 = local write "Valve V1 Open"(FALSE ("Valve V1 Open")) -> ()
